vi "DSP_conditioning_Rx.vi"(5 "rx.input valid":bool, 6 "rx.frequency shift":fxp<+/-,48,0> format="%#.48g", 7 "rx.reset":bool, 8 "rx.phase":fxp<+/-,21,0>, 10 "rx.impairments":T2={"inline gain I"=0.9999923706054688, "inline gain Q"=0.9999923706054688, "cross gain I"=0.0, "cross gain Q"=0.0, "pre-gain offset I"=0.0, "pre-gain offset Q"=0.0, "post-gain offset I"=0.0, "post-gain offset Q"=0.0}, 11 "data in":T1) -> (1 "rx.dsp reset done":bool, 2 "output valid":bool, 3 "data out":T1)   [LabVIEW 2017]
uses:
  <instrlib>/_niInstr/DSP/v1/Shared/Public/IQ Impairments.ctl
  <instrlib>/_niInstr/DSP/v1/Shared/Public/IQ Data.ctl
  <instrlib>/_niInstr/DSP/v1/FPGA/Public/Sub VIs/IQ Impairments/IQ Impairments - 1 spc.vi
  <instrlib>/_niInstr/DSP/v1/FPGA/Public/Sub VIs/Frequency Shift/Frequency Shift - 1 spc.vi
  <instrlib>/_niInstr/DSP/v1/FPGA/niInstr DSP v1 FPGA.lvlib
  <instrlib>/_niInstr/Basic Elements/v1/FPGA/niInstr Basic Elements v1 FPGA.lvlib
  <instrlib>/_niInstr/DSP/v1/FPGA/Public/Sub VIs/Fractional Interpolator/Fractional Interpolator - 1 spc - 2x oc.vi
  <instrlib>/_niInstr/DSP/v1/Shared/niInstr DSP v1 Shared.lvlib
panel:
  in  "rx.input sample rate":fxp<+,48,1>
  in  "rx.delay":fxp<+/-,18,0>
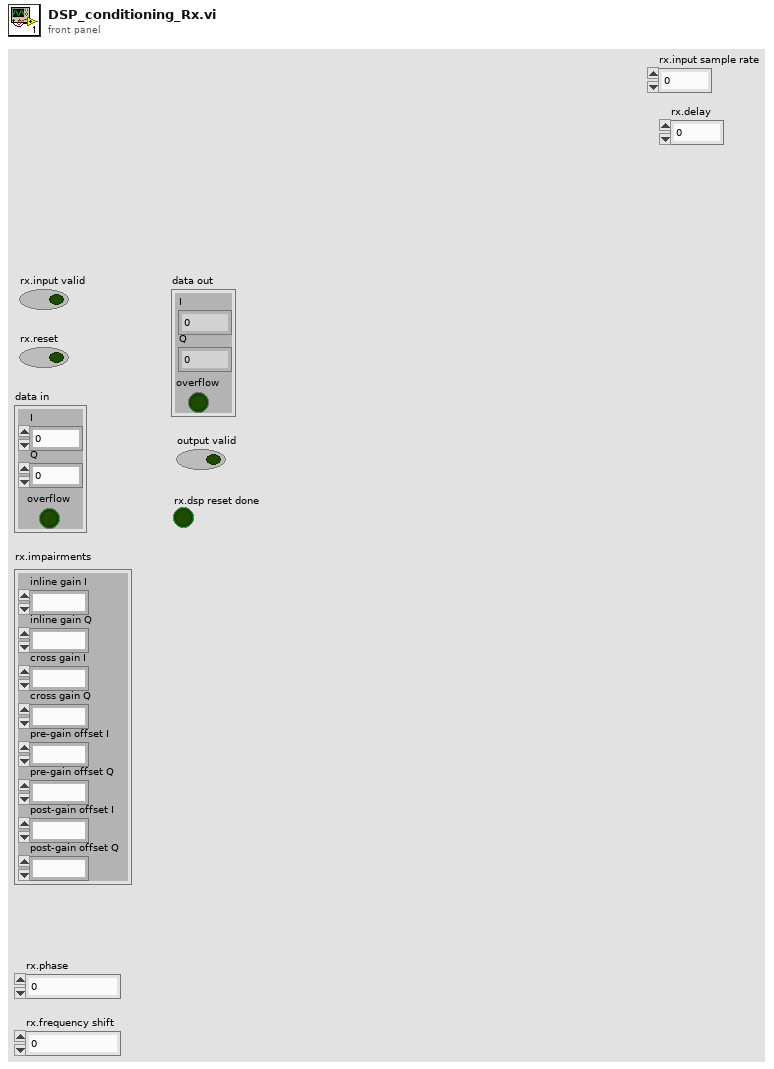
[diagram p1: front panel]
types:
  T1 = typedef "niInstr DSP v1 Shared.lvlib/IQ Data.ctl" = cluster{"I":fxp<+/-,18,1>, "Q":fxp<+/-,18,1>, "overflow":bool}
  T2 = typedef "niInstr DSP v1 Shared.lvlib/IQ Impairments.ctl" = cluster{"inline gain I":fxp<+/-,18,1>, "inline gain Q":fxp<+/-,18,1>, "cross gain I":fxp<+/-,18,1>, "cross gain Q":fxp<+/-,18,1>, "pre-gain offset I":fxp<+/-,18,1>, "pre-gain offset Q":fxp<+/-,18,1>, "post-gain offset I":fxp<+/-,18,1>, "post-gain offset Q":fxp<+/-,18,1>}
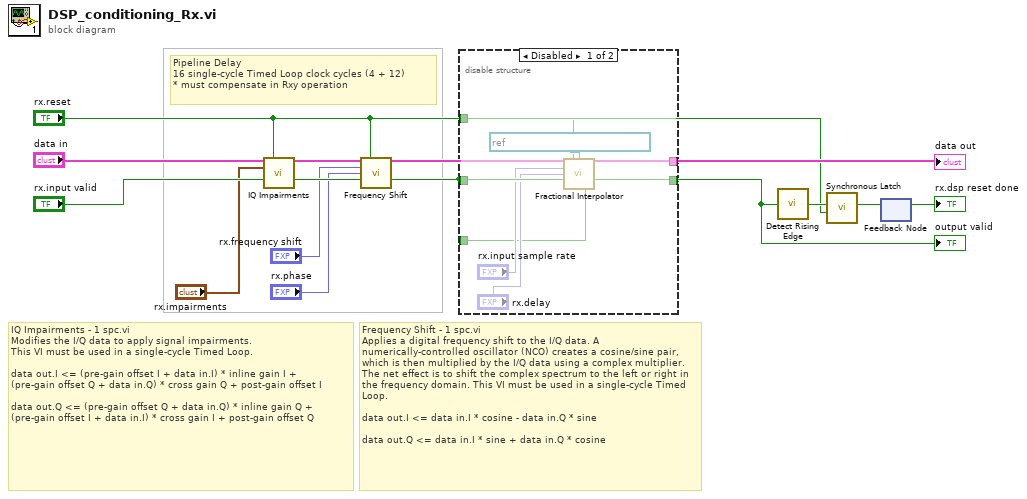
[diagram p0: block diagram]
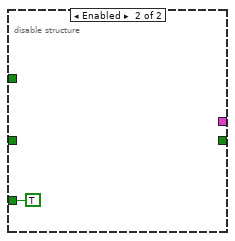
[diagram p2: hidden frame]
diagram:
  # "Frequency Shift - 1 spc.vi\nApplies a digital frequency shift to the I/Q data. A numerically-controlled oscillator (NCO) creates a cosine/sine pair, which is then multiplied by the I/Q data using a complex multiplier. The net effect is to shift the complex spectrum to the left or right in the frequency domain. This VI must be used in a single-cycle Timed Loop.\n\ndata out.I <= data in.I * cosine - data in.Q * sine\n\ndata out.Q <= data in.I * sine + data in.Q * cosine"
  # "IQ Impairments - 1 spc.vi\nModifies the I/Q data to apply signal impairments. \nThis VI must be used in a single-cycle Timed Loop.\n\ndata out.I <= (pre-gain offset I + data in.I) * inline gain I + \n(pre-gain offset Q + data in.Q) * cross gain Q + post-gain offset I\n\ndata out.Q <= (pre-gain offset Q + data in.Q) * inline gain Q +\n(pre-gain offset I + data in.I) * cross gain I + post-gain offset Q"
  # "Pipeline Delay \n16 single-cycle Timed Loop clock cycles (4 + 12)\n* must compensate in Rxy operation"
  n1 = call-poly <instrlib>:"IQ Impairments.vi"("data in"="data in", "reset"="rx.reset", "impairments"="rx.impairments", "input valid"="rx.input valid") -> ("data out"=w3:T1, "output valid"=w7:bool)  [unwired: 9 in, 1 out]
  n2 = call-poly <instrlib>:"Frequency Shift.vi"("data in"=w3, "reset"="rx.reset", "frequency shift"="rx.frequency shift", "phase"="rx.phase", "input valid"=w7) -> ("data out"=→"data out":T1, "output valid"=w1:bool)  [unwired: 8 in, 1 out]
  "output valid" <- w1
  n3 = disable-structure shown="Disabled" {
    disable-tunnel: [w21 _] -> _
    disable-tunnel: [w20 _] -> _
    disable-tunnel: w1 -> [w18 _]
    disable-tunnel: "rx.reset" -> [w15 _]
    disable-tunnel: [w14 TRUE ("signal")] -> _
    frame Disabled {
      n4 = call-poly <instrlib>:"Fractional Interpolator.vi"("reset"=w15, "clock x 2"=refnum<k21> "IO Module\\Data Clock x2", "input sample rate"="rx.input sample rate", "delay"="rx.delay", "input valid"=w18) -> ("data out"=w20:T1, "output valid"=w21:bool, "ready for input"=w14:bool)  [unwired: 7 in, 1 out]
    }
    frame Enabled {
    }
  }
  n5 = call <instrlib>:"Detect Rising Edge.vi"("signal"=w1) -> ("edge detected"=w9:bool)  [unwired: 14 in]
  n6 = call <instrlib>:"Synchronous Latch.vi"("clear"="rx.reset", "set"=w9) -> ("out"=w10:bool)  [unwired: 9 in]
  n7 = feedback #1() -> (→"rx.dsp reset done":bool)  [unwired: 1 in]
  n8 = feedback-in #1(w10) -> ()
